vi "bundleScanParameters.vi"(9 "Zoom":dbl[](array[numeric]), 10 "xyzNormalizedCoordinates":T1={"XYZ Start"=[{"X"=0.0, "Y"=0.0, "Z"=0.0}], "XYZ Stop"=[]}, 11 "AOL_Globals":T2={"Imaging Protocol"=enum."AOL Z-Stack", "Number of POI"=0, "Number of Miniscans"=0, "Number of Trials"=0, "Number of Cycles "=0, "# Averaged Frames"=0, "Laser power (%)"=0, "Pockels (V)"=0.0, "Acquisition Length (sec)"=0.0, "Fill time (us)"=0.0, "POI Dwell time (us)"=0.0, "Miniscan Dwell time per pixel (us)"=0.0, "PMT 1"=0.0, "PMT 2"=0.0, "Back Apperture (mA)"=200.0, "Frame Size"=0, "Center Frequency"=0.0, "Field of View (norm)"=0.0, "DwellTime (us)"=0.0, "Wavelength (nm)"=0.0, "Zoom"=0.0, "AOL Z"=0.0, "AOL Mode"=enum."Raster", "GridXY"=0.0, "GridZ"=0.0, "TriggerPeriod (sec)"=0.0, "Number of Pixels in Miniscan"=0, "Experiment folder path"=path "", "X centre"=0.0, "Y centre"=0.0, "Angle (degrees)"=0.0, "Plane Mode"=0, "Threshold"=[], "Regenerate Chirps"=FALSE, "Rectangle ROI length (pixels)"=0, "Rectangle ROI height (pixels)"=0, "AOD fill"=4900, "StartupDelay"=0, "Samples Wait after Trigger"=5080, "Slip Cycle"=600000, "Add Cycle"=TRUE, "Functional Mode"=enum."Point", "Z Start"=0.0, "Z Stop"=0.0, "# Planes"=0} {"Plane Mode" items=["XY Plane", "XZ Plane", "YZ Plane", "arbitraryplane"]; "Frame Size" items=["100X100"=100, "128X128"=128, "200X200"=200, "256X256"=256, "512X512"=512, "1024x1024"=1024, "2048x2048"=2048]; "Back Apperture (mA)" format="%#.6g"; "Pockels (V)" format="%#.6g"; "PMT 2" format="%#.6g"; "PMT 1" format="%#.6g"; "Angle (degrees)" format="%#.6g"; "POI Dwell time (us)" format="%#.6g"}) -> (1 "xyzImageStopNormalised":dbl[][](array[numeric]), 2 "xyzImageStartNormalised":dbl[][](array[numeric]), 3 "scanVariables":dbl[][](array[numeric]))   [LabVIEW 2017]
uses:
  Typedefs/Controls/AOL_Globals.ctl
  Typedefs/Imaging Protocols enum.ctl
  Typedefs/Frame Size.ctl
  Typedefs/AOL modes.ctl
  Typedefs/Plane Mode.ctl
  Typedefs/Functional Mode.ctl
  Global Variables/General Globals.vi
panel:
  out "FOV":dbl
  in  "Bypass with this manual value 2":bool caption="Bypass with this manual value"
  in  "Field of View":dbl
  out "size(s) 2":i32[](array[numeric])
  out "size":i32
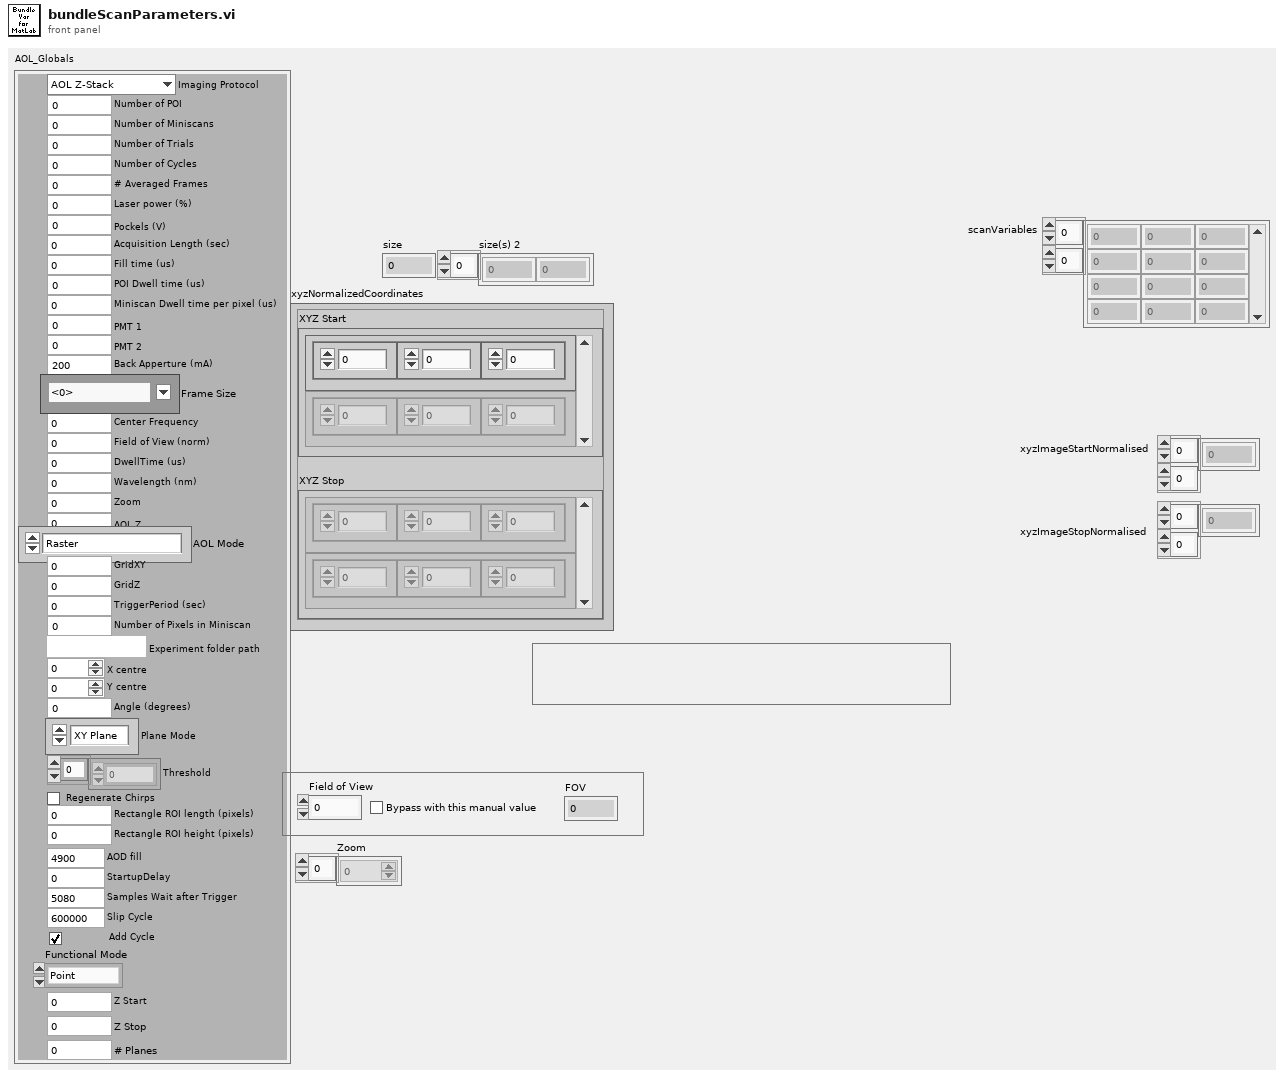
[diagram p1: front panel]
types:
  T1 = cluster{"XYZ Start":cluster{"X":sgl, "Y":sgl, "Z":sgl}[], "XYZ Stop":cluster{"X":sgl, "Y":sgl, "Z":sgl}[]}
  T2 = typedef "AOL_Globals.ctl" = cluster{"Imaging Protocol":T3, "Number of POI":u16, "Number of Miniscans":u16, "Number of Trials":u16, "Number of Cycles ":u64, "# Averaged Frames":u16, "Laser power (%)":u8, "Pockels (V)":dbl, "Acquisition Length (sec)":dbl, "Fill time (us)":dbl, "POI Dwell time (us)":dbl, "Miniscan Dwell time per pixel (us)":dbl, "PMT 1":dbl, "PMT 2":dbl, "Back Apperture (mA)":dbl, "Frame Size":T4, "Center Frequency":dbl, "Field of View (norm)":dbl, "DwellTime (us)":dbl, "Wavelength (nm)":dbl, "Zoom":dbl, "AOL Z":dbl, "AOL Mode":T5, "GridXY":dbl, "GridZ":dbl, "TriggerPeriod (sec)":dbl, "Number of Pixels in Miniscan":u16, "Experiment folder path":path, "X centre":dbl, "Y centre":dbl, "Angle (degrees)":dbl, "Plane Mode":T6, "Threshold":u16[], "Regenerate Chirps":bool, "Rectangle ROI length (pixels)":u16, "Rectangle ROI height (pixels)":u16, "AOD fill":u16, "StartupDelay":i32, "Samples Wait after Trigger":u16, "Slip Cycle":u32, "Add Cycle":bool, "Functional Mode":T7, "Z Start":dbl, "Z Stop":dbl, "# Planes":i32}
  T3 = typedef "Imaging Protocols enum.ctl" = enum16{"AOL Z-Stack", "Motor Z Stack", "Functional Acquisition", "Single Plane Acquisition", "Volume Acquisition", "Live Imaging", "Live Plane Imaging", "Live Volume Imaging"}
  T4 = typedef "Frame Size.ctl" = u16
  T5 = typedef "AOL modes.ctl" = enum16{"Raster", "Structural", "Pointing", "Mini Scan", "Alignment"}
  T6 = typedef "Plane Mode.ctl" = u16
  T7 = typedef "Functional Mode.ctl" = enum16{"Point", "Line", "Patch", "Plane", "Volume"}
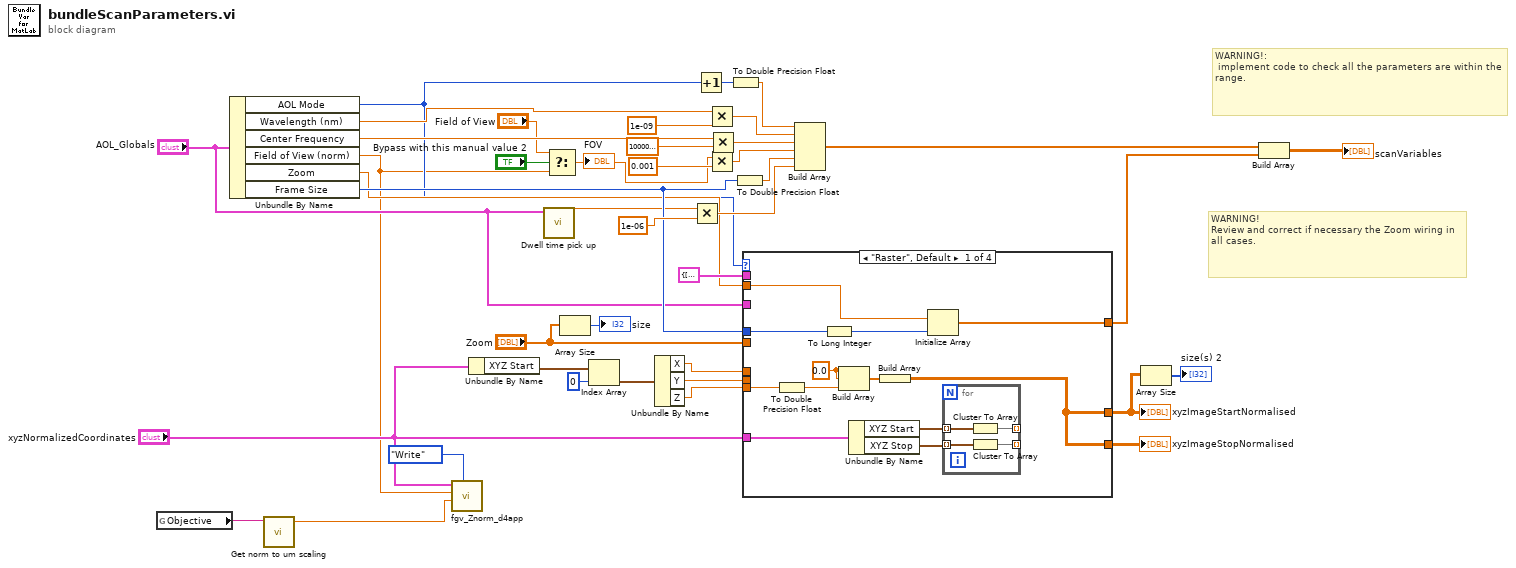
[diagram p0: block diagram]
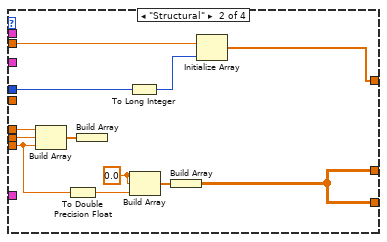
[diagram p2: hidden frame]
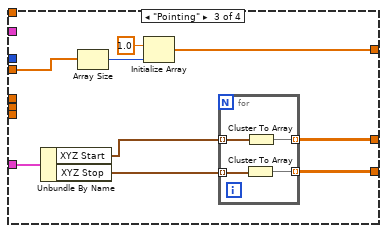
[diagram p3: hidden frame]
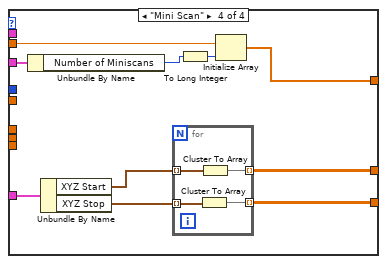
[diagram p4: hidden frame]
diagram:
  # "WARNING!\nReview and correct if necessary the Zoom wiring in all cases."
  # "WARNING!:\n implement code to check all the parameters are within the range."
  n1 = global read "General Globals.vi" "Objective"() -> (w3:string)
  n2 = Unbundle By Name("AOL_Globals") -> ("AOL Mode"=w6:T5, "Wavelength (nm)"=w41:dbl, "Center Frequency"=w31:dbl, "Field of View (norm)"=w1:dbl, "Zoom"=w18:dbl, "Frame Size"=w19:T4)
  n3 = call "Get norm to um scaling .vi"("Current Objective"=w3) -> ("Z_norm to um_scaling"=w2:dbl)  [unwired: 8 in, 2 out]
  n4 = call "fgv_Znorm_d4app.vi"("Function"=enum16{"Idle", "Write", "Read"}."Write", "Znorm_um_Scaling"=w2, "acceptance angle"=w1, "xyzNormalizedCoordinates"="xyzNormalizedCoordinates") -> ()  [unwired: 5 in, 3 out]
  n5 = Unbundle By Name("xyzNormalizedCoordinates") -> ("XYZ Start"=w25:cluster{"X":sgl, "Y":sgl, "Z":sgl}[])
  n6 = call "Dwell time pick up.vi"("AOL_Globals"="AOL_Globals") -> ("Dwell time (us)"=w14:dbl)  [unwired: 10 in]
  n7 = Select(t="Field of View", s="Bypass with this manual value 2", f=w1) -> (s? t:f=w13:dbl)
  "FOV" <- w13
  n8 = Array Size(array="Zoom") -> (size(s)=→"size":i32)
  n9 = Index Array(array=w25, index=0) -> (element=w24:cluster{"X":sgl, "Y":sgl, "Z":sgl})
  n10 = Unbundle By Name(w24) -> ("X"=w39:sgl, "Y"=w38:sgl, "Z"=w36:sgl)
  n11 = Multiply(x=w14, y=1e-06) -> (x*y=w29:dbl)
  n12 = Increment(x=w6) -> (x+1=w7:T5)
  n13 = Multiply(x=w41, y=1e-09) -> (x*y=w34:dbl)
  n14 = Multiply(x=w13, y=0.001) -> (x*y=w27:dbl)
  n15 = Multiply(x=w31, y=1000000.0) -> (x*y=w32:dbl)
  n16 = To Double Precision Float(number=w7) -> (double precision float=w40:dbl)
  n17 = To Double Precision Float(number=w19) -> (double precision float=w35:dbl)
  n18 = case shown="\"Raster\", Default" w6 {
    tunnel: w39 -> [_ w69 _ _]
    tunnel: w38 -> [_ w68 _ _]
    tunnel: "xyzNormalizedCoordinates" -> [w53 _ w78 w92]
    tunnel: T1 {"XYZ Start"=[{"X"=0.0, "Y"=0.0, "Z"=0.0}], "XYZ Stop"=[]} ("xyzNormalizedCoordinates") -> [_ _ _ _]
    tunnel: w36 -> [w44 w59 _ _]
    tunnel: [w42 w58 w76 w86] -> w16
    tunnel: [w42 w58 w70 w83] -> w22
    tunnel: w19 -> [w48 w65 _ _]
    tunnel: [w50 w66 w72 w88] -> w8
    tunnel: w18 -> [w49 w63 _ w89]
    tunnel: "Zoom" -> [_ _ w73 _]
    tunnel: "AOL_Globals" -> [_ _ _ w91]
    frame "Raster", Default {
      w45 = 0.0 ("element")
      n19 = To Double Precision Float(number=w44) -> (double precision float=w43:dbl)
      n20 = To Long Integer(number=w48) -> (32bit integer=w47:i32)
      n21 = Build Array(w45, w45, w43) -> (w46:dbl[])
      n22 = Unbundle By Name(w53) -> ("XYZ Start"=w52:cluster{"X":sgl, "Y":sgl, "Z":sgl}[], "XYZ Stop"=w51:cluster{"X":sgl, "Y":sgl, "Z":sgl}[])
      n23 = Build Array(w46) -> (w42:dbl[][])
      n24 = Initialize Array(w49, w47) -> (w50:dbl[])
      n25 = for {
        tunnel: w52 -> [w57] mode=indexing
        tunnel: [w56] -> _ mode=indexing
        tunnel: w51 -> [w55] mode=indexing
        tunnel: [w54] -> _ mode=indexing
        n26 = Cluster To Array(cluster=w57) -> (array=w56:sgl[])
        n27 = Cluster To Array(cluster=w55) -> (array=w54:sgl[])
      }
    }
    frame "Structural" {
      w61 = 0.0 ("element")
      n28 = Build Array(w69, w68, w59) -> (w67:sgl[])
      n29 = To Double Precision Float(number=w59) -> (double precision float=w60:dbl)
      n30 = Build Array(w67) -> ()  [unwired: 1 out]
      n31 = To Long Integer(number=w65) -> (32bit integer=w64:i32)
      n32 = Build Array(w61, w61, w60) -> (w62:dbl[])
      n33 = Build Array(w62) -> (w58:dbl[][])
      n34 = Initialize Array(w63, w64) -> (w66:dbl[])
    }
    frame "Pointing" {
      n35 = Unbundle By Name(w78) -> ("XYZ Start"=w77:cluster{"X":sgl, "Y":sgl, "Z":sgl}[], "XYZ Stop"=w71:cluster{"X":sgl, "Y":sgl, "Z":sgl}[])
      n36 = Array Size(array=w73) -> (size(s)=w75:i32)
      n37 = Initialize Array(1.0 ("element"), w75) -> (w72:dbl[])
      n38 = for {
        tunnel: w77 -> [w82] mode=indexing
        tunnel: [w81] -> w76 mode=indexing
        tunnel: w71 -> [w80] mode=indexing
        tunnel: [w79] -> w70 mode=indexing
        n39 = Cluster To Array(cluster=w80) -> (array=w79:sgl[])
        n40 = Cluster To Array(cluster=w82) -> (array=w81:sgl[])
      }
    }
    frame "Mini Scan" {
      n41 = Unbundle By Name(w91) -> ("Number of Miniscans"=w90:u16)
      n42 = Unbundle By Name(w92) -> ("XYZ Start"=w85:cluster{"X":sgl, "Y":sgl, "Z":sgl}[], "XYZ Stop"=w84:cluster{"X":sgl, "Y":sgl, "Z":sgl}[])
      n43 = for {
        tunnel: w85 -> [w96] mode=indexing
        tunnel: [w95] -> w86 mode=indexing
        tunnel: w84 -> [w94] mode=indexing
        tunnel: [w93] -> w83 mode=indexing
        n44 = Cluster To Array(cluster=w94) -> (array=w93:sgl[])
        n45 = Cluster To Array(cluster=w96) -> (array=w95:sgl[])
      }
      n46 = To Long Integer(number=w90) -> (32bit integer=w87:i32)
      n47 = Initialize Array(w89, w87) -> (w88:dbl[])
    }
  }
  "xyzImageStartNormalised" <- w16
  "xyzImageStopNormalised" <- w22
  n48 = Build Array(w40, w34, w32, w27, w35, w29) -> (w21:dbl[])
  n49 = Array Size(array=w16) -> (size(s)=→"size(s) 2":i32[])
  n50 = Build Array(w21, w8) -> (→"scanVariables":dbl[][])
